vi "Report Event.vi"(7 "Event Level (Info)":T1, 8 "error in (no error)":errorcluster, 10 "Message":string, 11 "LocalEventCollector in":refnum<class "LocalEventCollector.lvclass">) -> (0 "error out":errorcluster)   [LabVIEW 2020, in "Vecto.lvlib" / "LocalEventCollector.lvclass"]
uses:
  LocalEventCollector.lvclass
  Event Level.ctl
  LocalEventCollector.lvclass/LocalEventCollector.ctl
  lv-volatus/Volatus/Event Level.ctl
  lv-volatus/Volatus/Volatus.lvlib
  Event.ctl
  Vecto.lvlib
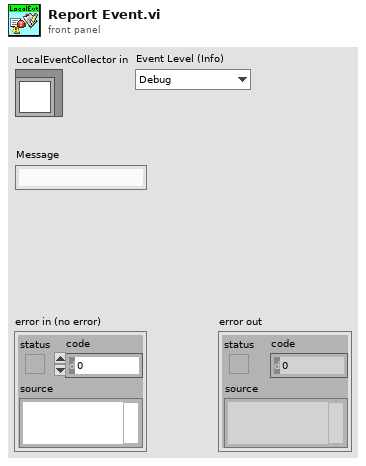
[diagram p1: front panel]
types:
  T1 = typedef "Vecto.lvlib/Event Level.ctl" = enum16{"Debug", "Info", "Warning", "Error"}
  T2 = typedef "Vecto.lvlib/LocalEventCollector.lvclass/Event.ctl" = cluster{"Time Stamp":timestamp, "Event Level":T3, "Message":string, "Error":errorcluster}
  T3 = typedef "Volatus.lvlib/Event Level.ctl" = enum16{"Debug", "Info", "Warning", "Error"}
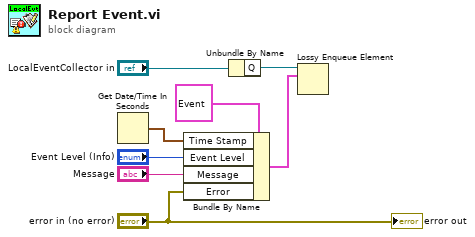
[diagram p0: block diagram]
diagram:
  n1 = Get Date/Time In Seconds() -> (seconds since 1Jan1904=w4:timestamp)
  n2 = Bundle By Name(cluster=T2 {"Time Stamp"=timestamp(0 s since 1904-01-01), "Event Level"=enum."Info", "Message"="", "Error"={"status"=FALSE, "code"=0, "source"=""}} ("Event"), "Time Stamp"=w4, "Event Level"="Event Level (Info)", "Message"="Message", "Error"="error in (no error)") -> (w1:T2)
  n3 = Unbundle By Name("LocalEventCollector in") -> ("Q"=w2:refnum<queue>)
  n4 = Lossy Enqueue Element(queue=w2, element=w1) -> ()  [unwired: 1 in, 4 out]
  "error out" <- "error in (no error)"
